vi "Send Voltage Settings.vi"(8 "error in (no error)":errorcluster, 11 "N5745A in":refnum<class "5745A.lvclass">) -> (0 "error out":errorcluster, 3 "N5745A out":refnum<class "5745A.lvclass">)   [LabVIEW 2018, in "5745A.lvlib" / "5745A.lvclass"]
doc: "This method is used to send the voltage setting to the N5745A Power Supply. It also calculates and sends the Over Voltage Protection (OVP) and Under Voltage Limit (UVL) setting values.\n\nNote: During development, it was observed that although the instrument does not allow OVP and UVL outside the +/-5% range from nominal setting, using exactly this +/- 5% range may pose errors, potentially due to internal instrument digit rounding. The +/- 6% range provides settings less proned to errors for this instrument. This is the reason why the nominal voltage is multplied by 0.94 and 1.06 to calculate UVL and OVP, respectively, in the the block diagram."
uses:
  5745A.lvclass
  builds/Power_Supply.lvlibp/Power Supply.lvclass
  C:/Users/Ron.Dexter.LUMINARTECH/Desktop/builds/Power_Supply.lvlibp/Power Supply.lvclass
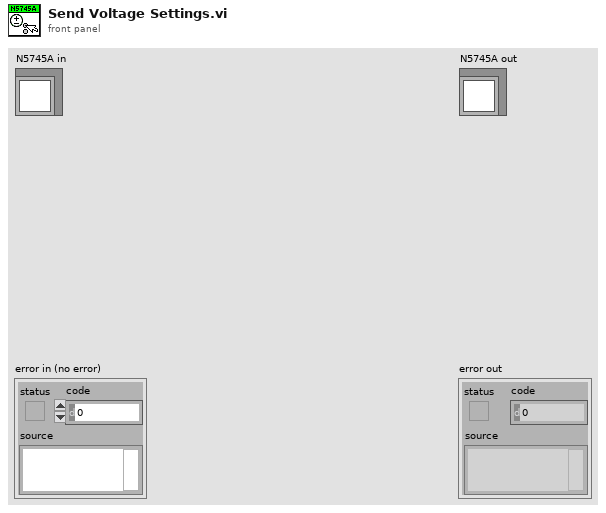
[diagram p1: front panel]
types:
  T1 = typedef "Power_Supply.lvlibp/Supply Settings.ctl" = cluster{"Voltage":dbl, "Current":dbl, "Output":bool}
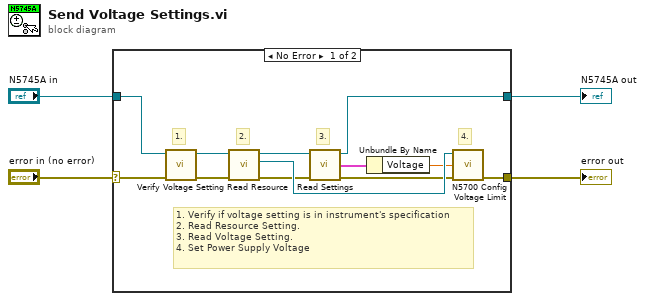
[diagram p0: block diagram]
diagram:
  n1 = case shown="No Error" "error in (no error)" {
    selector: "error in (no error)" -> [w13 w18]
    tunnel: [w15 w18] -> w3
    tunnel: [w8 w17] -> w1
    tunnel: "N5745A in" -> [w14 w17]
    frame No Error {
      # "4."
      # "2."
      # "1."
      # "1. Verify if voltage setting is in instrument's specification\n2. Read Resource Setting.\n3. Read Voltage Setting.\n4. Set Power Supply Voltage"
      # "3."
      n2 = call "Verify Voltage Setting.vi"("error in (no error)"=w13, "N5745A in"=w14) -> ("error out"=w12:errorcluster, "N5745A out"=w11:refnum<class "5745A.lvclass">)  [unwired: 8 in]
      n3 = call "Read Resource.vi"("error in"=w12, "Power Supply in"=w11) -> ("error out"=w6:errorcluster, "Resource"=w16:refnum<visa-resource-name>, "Power Supply out"=w9:refnum<class "5745A.lvclass">)  [unwired: 7 in]
      n4 = call "Read Settings.vi"("error in (no error)"=w6, "Power Supply in"=w9) -> ("error out"=w5:errorcluster, "Settings"=w10:T1, "Power Supply out"=w8:refnum<class "5745A.lvclass">)  [unwired: 7 in]
      n5 = Unbundle By Name(w10) -> ("Voltage"=w7:dbl)
      n6 = call <instrlib>:"N5700 Config Voltage Limit.vi"("error"=w5, "Volt Limit"=w7, "VISA"=w16) -> ("error out"=w15:errorcluster)  [unwired: 4 in, 1 out]
    }
    frame Error {
    }
  }
  "error out" <- w3
  "N5745A out" <- w1
